vi "Draw Mean.vi"(7 "Auto Defer Panel Updates? (T)":bool=TRUE, 8 "error in (no error)":errorcluster, 11 "Graph Manager in":refnum<class "Graph Manager.lvclass">) -> (0 "error out":errorcluster, 3 "Graph Manager out":refnum<class "Graph Manager.lvclass">)   [LabVIEW 2016, in "Graph Manager.lvclass"]
uses:
  Graph Manager.lvclass
  Graph Manager.lvclass/Graph Manager.ctl
  comm/nan operations/nan operations.lvlib
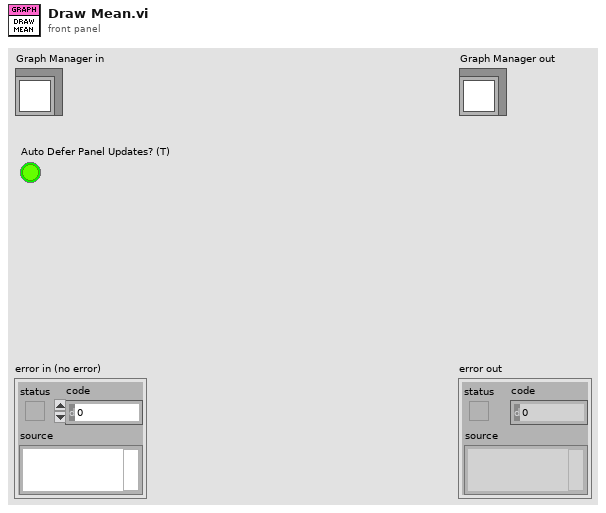
[diagram p1: front panel]
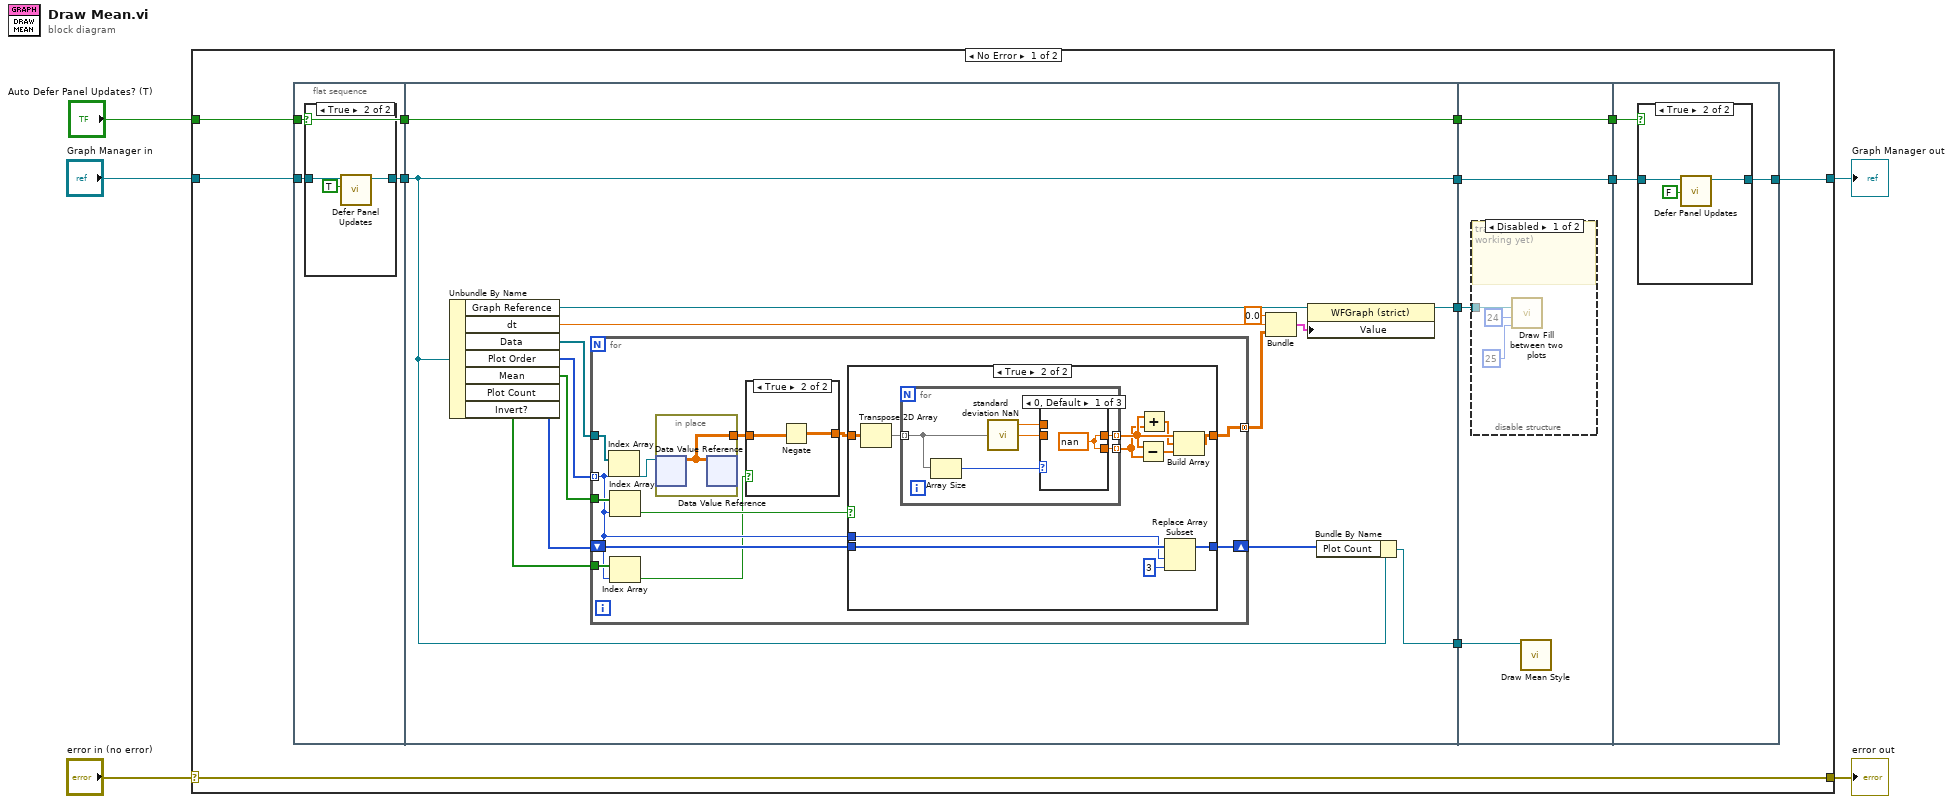
[diagram p0: block diagram]
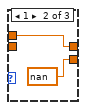
[diagram p5: hidden frame]
diagram:
  n1 = case shown="No Error" "error in (no error)" {
    selector: "error in (no error)" -> [w17 w95]
    tunnel: [w17 w95] -> w4
    tunnel: [w14 w94] -> w2
    tunnel: "Graph Manager in" -> [w16 w94]
    tunnel: "Auto Defer Panel Updates? (T)" -> [w9 _]
    frame No Error {
      n2 = flat-sequence {
        tunnel: w16 -> [w20]
        tunnel: [w19] -> w15
        tunnel: w9 -> [w18]
        tunnel: [w18] -> w6
        tunnel: w15 -> [w29]
        tunnel: [w29] -> w13
        tunnel: [w32] -> w11
        tunnel: [w27] -> w10
        tunnel: [w25] -> w7
        tunnel: w6 -> [w25]
        tunnel: w13 -> [w83]
        tunnel: [w83] -> w12
        tunnel: w11 -> [w82]
        tunnel: w10 -> [w81]
        tunnel: [w80] -> w8
        tunnel: w7 -> [w80]
        tunnel: w12 -> [w89]
        tunnel: [w88] -> w14
        tunnel: w8 -> [w87]
        frame #0 {
          n3 = case shown="True" w18 {
            tunnel: w20 -> [w21 w24]
            tunnel: [w21 w23] -> w19
            frame False {
            }
            frame True {
              n4 = call-dynamic "Defer Panel Updates.vi"("Defer Panel Updates"=TRUE, "Graph Manager in"=w24) -> ("Graph Manager out"=w23:refnum<class "Graph Manager.lvclass">)  [unwired: 8 in, 1 out]
            }
          }
        }
        frame #1 {
          n5 = Unbundle By Name(w29) -> ("Graph Reference"=w33:refnum<vi>, "dt"=w36:dbl, "Data"=w38:refnum<data-value>[], "Plot Order"=w39:i32[], "Mean"=w31:bool[], "Plot Count"=w30:i32[], "Invert?"=w26:bool[])
          n6 = for {
            tunnel: [w49] -> w37 mode=concatenating
            tunnel: w38 -> [w51]
            tunnel: w39 -> [w43] mode=indexing
            tunnel: w31 -> [w48]
            shift-right: [w46] -> w28
            shift-left: w30 -> [w45]
            tunnel: w26 -> [w44]
            n7 = Index Array(array=w51, index=w43) -> (element=w50:refnum<data-value>)
            n8 = Index Array(array=w48, index=w43) -> (element=w47:bool)
            n9 = Index Array(array=w44, index=w43) -> (element=w42:bool)
            n10 = in-place {
              in-place-border: [w79] -> w41
              n11 = in-place-dvr #1(w50) -> (w79:dbl[][])  [unwired: 1 out]
              n12 = in-place-dvr #1(w79) -> ()  [unwired: 2 out]
            }
            n13 = case shown="True" w42 {
              tunnel: w41 -> [w52 w54]
              tunnel: [w52 w53] -> w40
              frame False {
              }
              frame True {
                n14 = Negate(x=w54) -> (-x=w53:dbl[][])
              }
            }
            n15 = case shown="True" w47 {
              tunnel: w40 -> [w56 w67]
              tunnel: [w56 w65] -> w49
              tunnel: [w55 w60] -> w46
              tunnel: w45 -> [w55 w59]
              tunnel: w43 -> [_ w58]
              frame False {
              }
              frame True {
                n16 = Transpose 2D Array(2D array=w67) -> (transposed array=w66:dbl[][])
                n17 = for {
                  tunnel: w66 -> [w73] mode=indexing
                  tunnel: [w69] -> w64 mode=indexing
                  tunnel: [w68] -> w63 mode=indexing
                  n18 = Array Size(array=w73) -> (size(s)=w72:i32)
                  n19 = call "standard deviation NaN.vi"("Array"=w73) -> ("standard deviation"=w70:dbl, "mean"=w71:dbl)  [unwired: 2 in, 1 out]
                  n20 = case shown="0, Default" w72 {
                    tunnel: w71 -> [_ w75 w78]
                    tunnel: w70 -> [_ _ w77]
                    tunnel: [w74 w75 w78] -> w69
                    tunnel: [w74 nan w77] -> w68
                    frame 0, Default {
                      w74 = nan
                    }
                    frame 1 {
                    }
                    frame 2.. {
                    }
                  }
                }
                n21 = Subtract(x=w64, y=w63) -> (x-y=w61:dbl[])
                n22 = Add(x=w64, y=w63) -> (x+y=w62:dbl[])
                n23 = Replace Array Subset(array=w59, new element=3 ("new element/subarray"), index=w58) -> (w60:i32[])
                n24 = Build Array(w64, w62, w61) -> (w65:dbl[][])
              }
            }
          }
          n25 = Bundle(0.0, "dt"=w36, "Impulse Data"=w37) -> (w34:cluster{dbl, "dt":dbl, "Impulse Data":dbl[][]})  [unwired: 1 in]
          n26 = property class="WFGraph (strict)"(reference=w33, "Value"=w34) -> (reference out=w32:refnum<vi>)  [unwired: 1 in, 1 out]
          n27 = Bundle By Name(cluster=w29, "Plot Count"=w28) -> (w27:refnum<class "Graph Manager.lvclass">)
        }
        frame #2 {
          n28 = disable-structure shown="Disabled" {
            disable-tunnel: w82 -> [w86 _]
            frame Disabled {
              # "transparent fill (not working yet)"
              n29 = call "Draw Fill between two plots.vi"("Bottom Line"=u32 25, "Top Line"=u32 24, "Graph Reference"=w86) -> ()  [unwired: 9 in]
            }
            frame Enabled {
            }
          }
          n30 = call-dynamic "Draw Mean Style.vi"("Graph Manager in"=w81) -> ()  [unwired: 9 in, 2 out]
        }
        frame #3 {
          n31 = case shown="True" w87 {
            tunnel: w89 -> [w90 w93]
            tunnel: [w90 w92] -> w88
            frame False {
            }
            frame True {
              n32 = call-dynamic "Defer Panel Updates.vi"("Defer Panel Updates"=FALSE, "Graph Manager in"=w93) -> ("Graph Manager out"=w92:refnum<class "Graph Manager.lvclass">)  [unwired: 8 in, 1 out]
            }
          }
        }
      }
    }
    frame Error {
    }
  }
  "error out" <- w4
  "Graph Manager out" <- w2
